vi "read_sync_num.vi"() -> (3 "return":u32)   [LabVIEW 2011]
uses:
  canopen_dll_master.dll
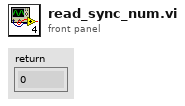
[diagram p1: front panel]
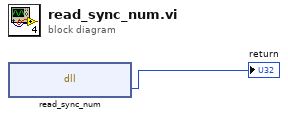
[diagram p0: block diagram]
diagram:
  n1 = dll-call lib="canopen_dll_master.dll" fn="read_sync_num"() -> ("return type"=→"return":u32)  [unwired: 3 in, 2 out]
